vi "CarWash_Controller.vi"(8 "error in":errorcluster) -> (0 "error out":errorcluster)   [LabVIEW 2019]
uses:
  #typedef_Queue_enum.ctl
  #typedef_Controller_Action_enum.ctl
  #typedef_Data_Controller.ctl
  #typedef_EntryConsole_Action_enum.ctl
  #typedef_WashDisplay_Action_enum.ctl
  #typedef_VehiclePosition_Action_enum.ctl
  #typedef_Data_Entry.ctl
  #typedef_Data_Cluster.ctl
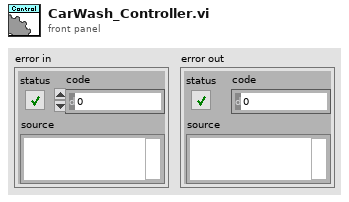
[diagram p1: front panel]
types:
  T1 = typedef "#typedef_Queue_enum.ctl" = enum16{"ERROR_default", "Obtain", "Enqueue", "GetStatus", "Flush", "Release"}
  T2 = typedef "#typedef_Data_Controller.ctl" = cluster{"EntryConsole_Action":T3, "WashDisplay_Action":T4, "Controller_Action":T5, "VehiclePosition_Action":T6}
  T3 = typedef "#typedef_EntryConsole_Action_enum.ctl" = enum16{"Init", "ERROR_DEFAULT", "Idle", "Pending_Wash_Cycle", "Clear_Console", "Close", "Error_Handler", "Exit"}
  T4 = typedef "#typedef_WashDisplay_Action_enum.ctl" = enum16{"Init", "ERROR_DEFAULT", "Idle", "Specific", "Close", "Error_Handler", "Exit"}
  T5 = typedef "#typedef_Controller_Action_enum.ctl" = enum16{"Init", "ERROR_DEFAULT", "Idle", "Read database", "Close", "Error_Handler", "Exit"}
  T6 = typedef "#typedef_VehiclePosition_Action_enum.ctl" = enum16{"Init", "ERROR_DEFAULT", "Idle", "Specific", "Close", "Error_Handler", "Exit"}
  T7 = typedef "#typedef_Data_Cluster.ctl" = cluster{"Dummy":dbl, "EntryConsole_Action":T3, "WashDisplay_Action":T4, "Controller_Action":T5, "VehiclePosition_Action":T6}
  T8 = typedef "#typedef_Data_Entry.ctl" = cluster{"Under Body Wash":bool, "Bug Remover":bool, "Pre-Soak":bool, "High Pressure Wash (default)":bool, "Low Pressure Wax":bool, "Spot Free Rinse":bool, "Tire Shine Foam":bool, "Air Dry":bool, "Start":bool, "EntryConsole_Action":T3}
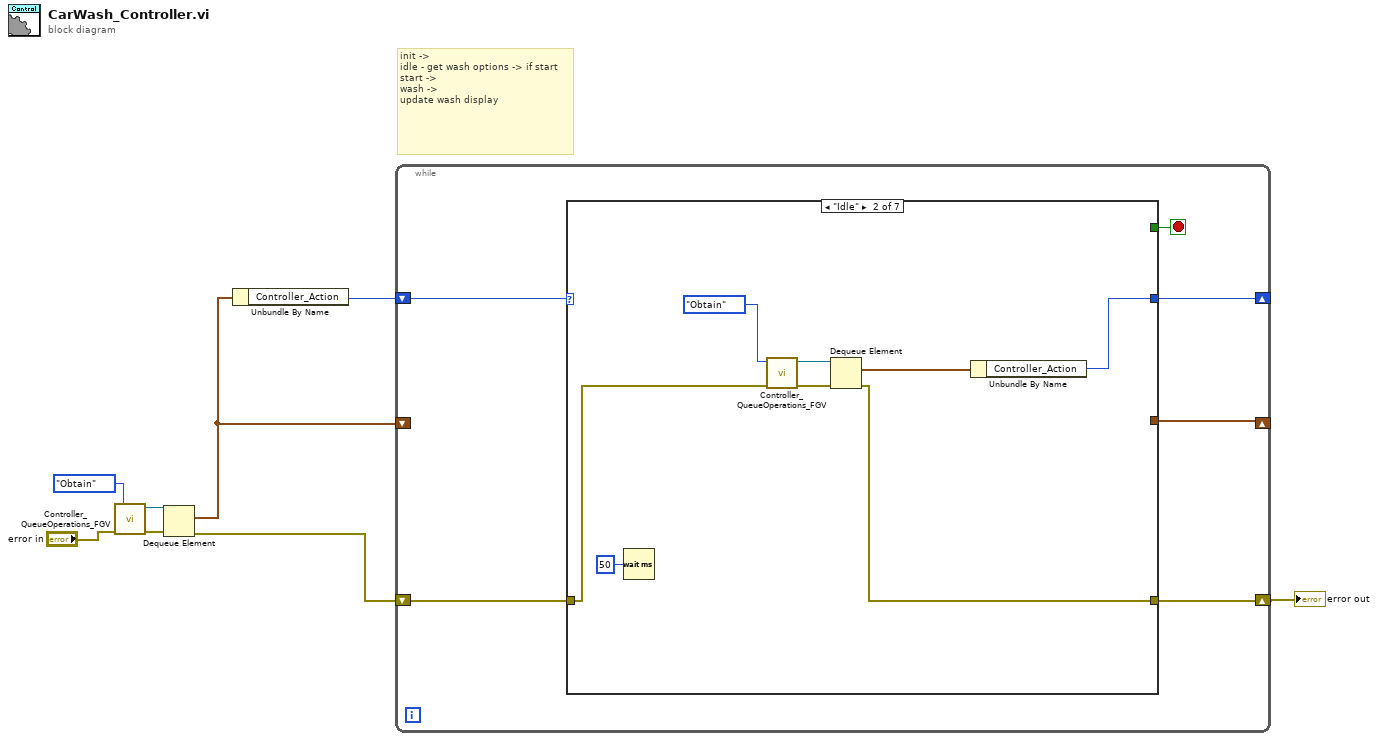
[diagram p0: block diagram]
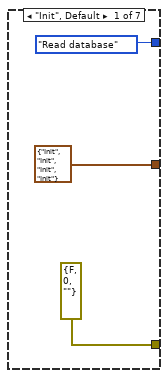
[diagram p2: hidden frame]
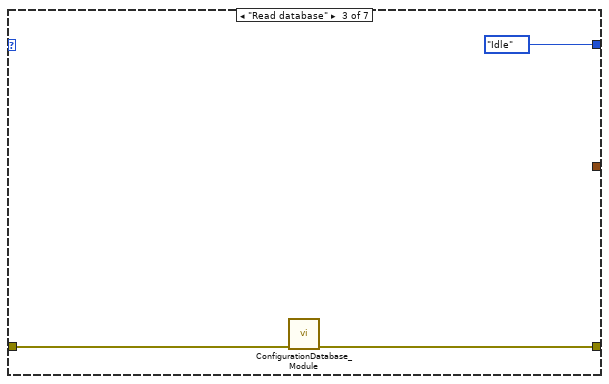
[diagram p3: hidden frame]
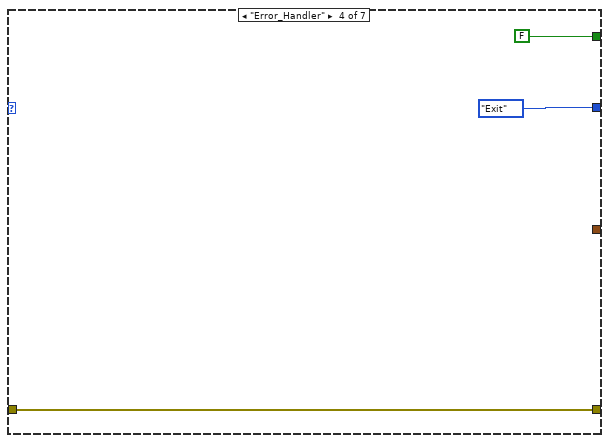
[diagram p4: hidden frame]
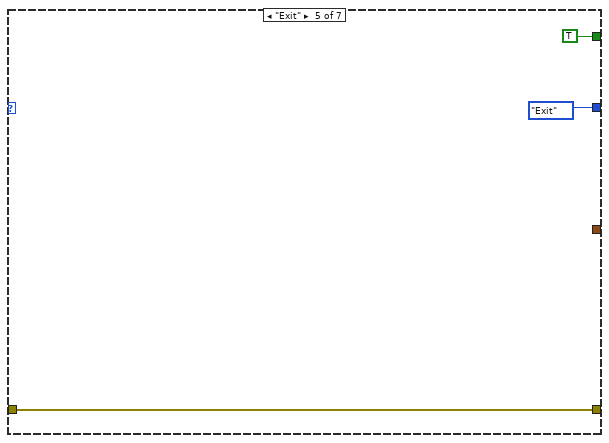
[diagram p5: hidden frame]
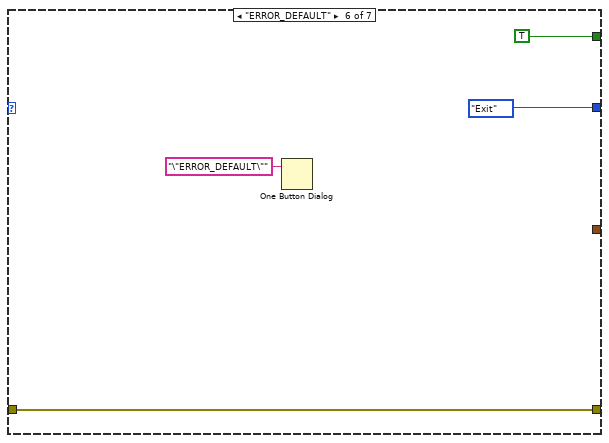
[diagram p6: hidden frame]
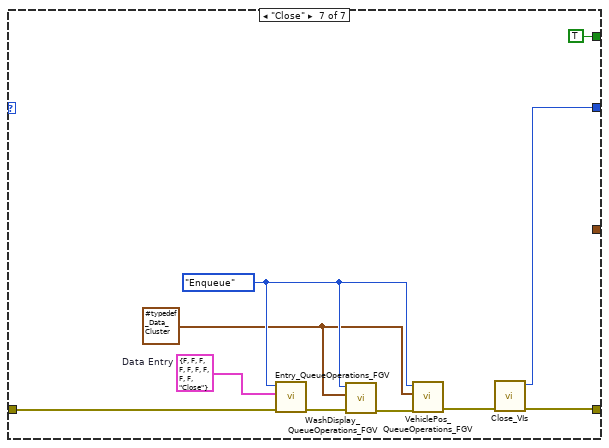
[diagram p7: hidden frame]
diagram:
  # "init ->\nidle - get wash options -> if start\nstart ->\nwash ->\nupdate wash display"
  n1 = call "Controller_QueueOperations_FGV.vi"("error in"="error in", "Action"=#typedef_Queue_enum."Obtain") -> ("error out"=w3:errorcluster, "queue ref"=w2:refnum<queue>)  [unwired: 6 in, 2 out]
  n2 = Dequeue Element(queue=w2, error in (no error)=w3) -> (element=w4:T2, error out=w6:errorcluster)  [unwired: 1 in, 2 out]
  n3 = Unbundle By Name(w4) -> ("Controller_Action"=w5:T5)
  n4 = while {
    shift-right: [w11] -> _
    shift-left: w5 -> [w14]
    shift-right: [w9] -> _
    shift-left: w4 -> [_]
    shift-right: [w10] -> w1
    shift-left: w6 -> [w12]
    stop <- w13 stop-if-true
    n5 = case shown="\"Idle\"" w14 {
      tunnel: [_ _ _ FALSE TRUE TRUE TRUE] -> w13
      tunnel: w12 -> [_ w24 w28 w30 w33 w36 w48]
      tunnel: [errorcluster {"status"=FALSE, "code"=0, "source"=""} ("error constant") w20 w26 w30 w33 w36 w42] -> w10
      tunnel: [#typedef_Controller_Action_enum."Read database" ("Enum") w22 #typedef_Controller_Action_enum."Idle" ("Enum") #typedef_Controller_Action_enum."Exit" ("Enum") #typedef_Controller_Action_enum."Exit" ("Enum") #typedef_Controller_Action_enum."Exit" ("Enum") w41] -> w11
      tunnel: [T2 {"EntryConsole_Action"=enum."Init", "WashDisplay_Action"=enum."Init", "Controller_Action"=enum."Init", "VehiclePosition_Action"=enum."Init"} ("Data") _ _ _ _ _ _] -> w9
      frame "Init", Default {
      }
      frame "Idle" {
        n6 = Wait (ms)(milliseconds to wait=u32 50) -> ()  [unwired: 1 out]
        n7 = call "Controller_QueueOperations_FGV.vi"("error in"=w24, "Action"=#typedef_Queue_enum."Obtain") -> ("error out"=w21:errorcluster, "queue ref"=w18:refnum<queue>)  [unwired: 6 in, 2 out]
        n8 = Dequeue Element(queue=w18, error in (no error)=w21) -> (element=w23:T2, error out=w20:errorcluster)  [unwired: 1 in, 2 out]
        n9 = Unbundle By Name(w23) -> ("Controller_Action"=w22:T5)
      }
      frame "Read database" {
        n10 = call "ConfigurationDatabase_Module.vi"("error in"=w28) -> ("error out"=w26:errorcluster)  [unwired: 9 in, 1 out]
      }
      frame "Error_Handler" {
      }
      frame "Exit" {
      }
      frame "ERROR_DEFAULT" {
        n11 = One Button Dialog(message="\"ERROR_DEFAULT\"") -> ()  [unwired: 1 in, 1 out]
      }
      frame "Close" {
        w39 = T7 {"Dummy"=0.0, "EntryConsole_Action"=enum."Init", "WashDisplay_Action"=enum."Init", "Controller_Action"=enum."Init", "VehiclePosition_Action"=enum."Init"} ("Data")
        w40 = T8 {"Under Body Wash"=FALSE, "Bug Remover"=FALSE, "Pre-Soak"=FALSE, "High Pressure Wash (default)"=FALSE, "Low Pressure Wax"=FALSE, "Spot Free Rinse"=FALSE, "Tire Shine Foam"=FALSE, "Air Dry"=FALSE, "Start"=FALSE, "EntryConsole_Action"=enum."Close"}  # Data Entry
        w45 = #typedef_Queue_enum."Enqueue" ("Action")
        n12 = call "Entry_QueueOperations_FGV.vi"("error in"=w48, "Data"=w40, "Action"=w45) -> ("error out"=w47:errorcluster)  [unwired: 5 in, 3 out]
        n13 = call "WashDisplay_QueueOperations_FGV.vi"("error in"=w47, "Data"=w39, "Action"=w45) -> ("error out"=w46:errorcluster)  [unwired: 5 in, 3 out]
        n14 = call "VehiclePos_QueueOperations_FGV.vi"("error in"=w46, "Data"=w39, "Action"=w45) -> ("error out"=w43:errorcluster)  [unwired: 5 in, 3 out]
        n15 = call "Close_VIs.vi"("error in"=w43) -> ("error out"=w42:errorcluster, "State Out"=w41:T5)  [unwired: 9 in]
      }
    }
  }
  "error out" <- w1
